vi "SRV_JPEG Filepath_Movie.vi"(1 "Count":i32, 2 "Dir path for JPEG file":path, 5 "Timestamp String":string) -> (7 "JPEG Filepath":path)   [LabVIEW 2014]
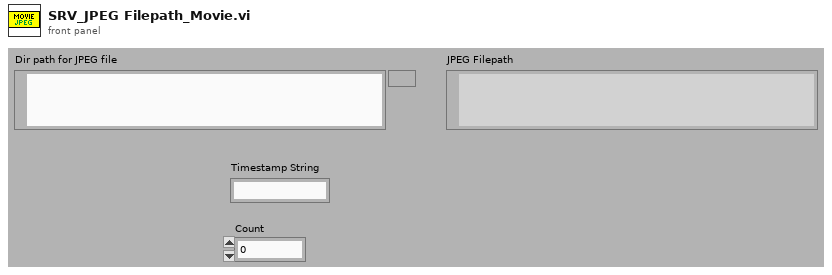
[diagram p1: front panel]
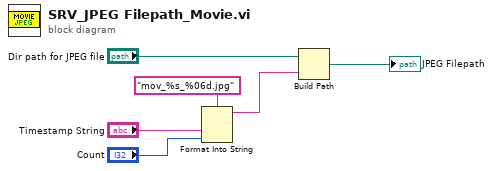
[diagram p0: block diagram]
diagram:
  n1 = Format Into String(format string="mov_%s_%06d.jpg", "Timestamp String", "Count") -> (resulting string=w3:string)  [unwired: 2 in, 1 out]
  n2 = Build Path(base path="Dir path for JPEG file", name or relative path=w3) -> (appended path=→"JPEG Filepath":path)
